vi "欧姆龙PLC通讯Fans UDP-写PLC寄存器编码.vi"(10 "数据":dbl[](array[numeric]), 11 "起始地址16":string) -> (3 "写入数据编码":string)   [LabVIEW 2014]
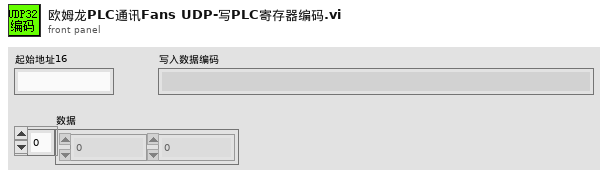
[diagram p1: front panel]
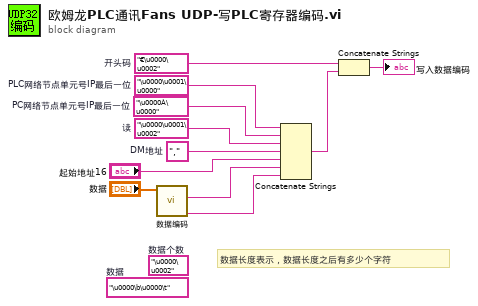
[diagram p0: block diagram]
diagram:
  w8 = "\u0000À\u0000"  # PC网络节点单元号IP最后一位
  w7 = "\u0000\u0001\u0000"  # PLC网络节点单元号IP最后一位
  w6 = "€\u0000\u0002"  # 开头码
  (unwired) "\u0000\b\u0000\t"  # 数据
  (unwired) "\u0000\u0002"  # 数据个数
  w3 = "‚"  # DM地址
  w2 = "\u0000\u0001\u0002"  # 读
  # "数据长度表示，数据长度之后有多少个字符"
  n1 = call "数据编码.vi"("数据"="数据") -> ("字符串"=w1:string, "16bit寄存器个数"=w10:string)  [unwired: 9 in]
  n2 = Concatenate Strings(w7, w8, w2, w3, "起始地址16", w10, w1) -> (w9:string)
  n3 = Concatenate Strings(w6, w9) -> (→"写入数据编码":string)
